vi "libssh2_crypto_engine.vi"(8 "error in (no error)":errorcluster) -> (0 "error out":errorcluster, 2 "crypto engine":T1(ring))   [LabVIEW 2013, in "libssh2.lvlib"]
doc: "Get the crypto engine used by libssh2."
uses:
  libssh2.lvlib
  Global Settings.vi
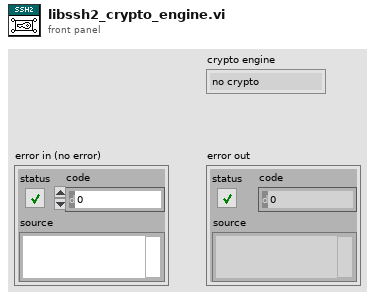
[diagram p1: front panel]
types:
  T1 = enum16{"no crypto", "OpenSSL", "gcrypt", "mbedTLS", "WinCNG", "OS400qc3"}
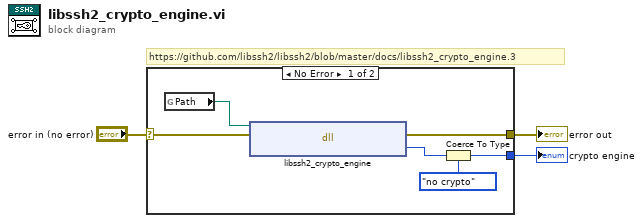
[diagram p0: block diagram]
diagram:
  # "https://github.com/libssh2/libssh2/blob/master/docs/libssh2_crypto_engine.3"
  n1 = case shown="No Error" "error in (no error)" {
    selector: "error in (no error)" -> [w7 w10]
    tunnel: [w8 w10] -> w3
    tunnel: [w5 _] -> w1
    frame No Error {
      n2 = global read "Global Settings.vi" "Path"() -> (w9:path)
      n3 = dll-call lib="?" fn="libssh2_crypto_engine"(path in=w9, error in=w7) -> (error out=w8:errorcluster, "return value"=w6:i32)  [unwired: 1 in, 1 out]
      n4 = Coerce To Type(0:w6, 1:T1."no crypto" ("crypto engine")) -> (2:w5:T1)
    }
    frame Error {
    }
  }
  "error out" <- w3
  "crypto engine" <- w1
